vi "Version.vi"(0 "VISA Resource Name":refnum<visa-resource-name>, 11 "error in (no error)":errorcluster) -> (2 "Module 3":string, 3 "Measurement Processor":string, 4 "VISA Resource Name Out":refnum<visa-resource-name>, 6 "I/O Processor":string, 8 "Front Panel Processor":string, 10 "Module 2":string, 13 "Module 1":string, 14 "SCPI Version":string, 15 "error out":errorcluster)   [LabVIEW 2012, in "Agilent 34970.lvlib"]
doc: "This VI queries the HP34970A as well as all its modules for version information."
uses:
  <instrlib>/Agilent 34970/Agilent 34970.lvlib
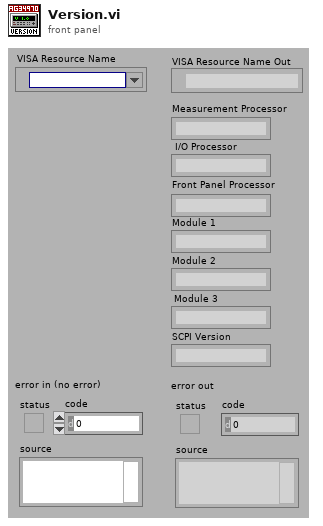
[diagram p1: front panel]
types:
  T1 = cluster{"[0]":string, "[1]":string, "[2]":string, "[3]":string, "[4]":string}
  T2 = cluster{"Output String Array[0]":string, "Output String Array[1]":string, "Output String Array[2]":string}
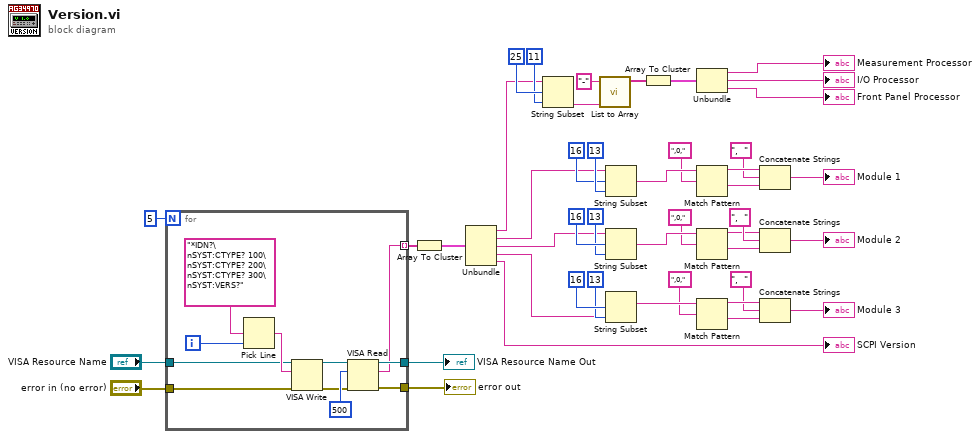
[diagram p0: block diagram]
diagram:
  n1 = for {
    N: 5 -> [_]
    tunnel: [w52] -> w43
    tunnel: [w51] -> w42
    tunnel: "VISA Resource Name" -> [w49]
    tunnel: "error in (no error)" -> [w48]
    tunnel: [w46] -> w7 mode=indexing
    i -> [w55]
    n2 = Pick Line(multi-line string="*IDN?\nSYST:CTYPE? 100\nSYST:CTYPE? 200\nSYST:CTYPE? 300\nSYST:VERS?", line index=w55) -> (output string=w50:string)  [unwired: 1 in]
    n3 = VISA Write(VISA resource name=w49, write buffer=w50, error in (no error)=w48) -> (VISA resource name out=w53:refnum<visa-resource-name>, error out=w47:errorcluster)  [unwired: 1 out]
    n4 = VISA Read(VISA resource name=w53, byte count=u32 500 ("byte count (0)"), error in (no error)=w47) -> (VISA resource name out=w51:refnum<visa-resource-name>, read buffer=w46:string, error out=w52:errorcluster)  [unwired: 1 out]
  }
  "VISA Resource Name Out" <- w42
  "error out" <- w43
  n5 = Array To Cluster(array=w7) -> (cluster=w6:T1)
  n6 = Unbundle(w6) -> ("[0]"=w2:string, "[1]"=w5:string, "[2]"=w4:string, "[3]"=w1:string, "[4]"=→"SCPI Version":string)
  n7 = String Subset(string=w2, offset (0)=25, length (rest)=11 ("length")) -> (substring=w23:string)
  n8 = call <instrlib>:"List to Array.vi"("List (empty)"=w23, "Separator (,)"="-" ("Separator")) -> ("Output String Array"=w41:string[])  [unwired: 8 in, 1 out]
  n9 = String Subset(string=w5, offset (0)=16, length (rest)=13 ("length")) -> (substring=w30:string)
  n10 = String Subset(string=w4, offset (0)=16, length (rest)=13 ("length")) -> (substring=w34:string)
  n11 = String Subset(string=w1, offset (0)=16, length (rest)=13 ("length")) -> (substring=w39:string)
  n12 = Array To Cluster(array=w41) -> (cluster=w22:T2)
  n13 = Unbundle(w22) -> ("Output String Array[0]"=→"Measurement Processor":string, "Output String Array[1]"=→"I/O Processor":string, "Output String Array[2]"=→"Front Panel Processor":string)
  n14 = Match Pattern(string=w30, regular expression=",0," ("string")) -> (before substring=w27:string, after substring=w28:string)  [unwired: 1 in, 2 out]
  n15 = Match Pattern(string=w34, regular expression=",0," ("string")) -> (before substring=w32:string, after substring=w35:string)  [unwired: 1 in, 2 out]
  n16 = Match Pattern(string=w39, regular expression=",0," ("string")) -> (before substring=w37:string, after substring=w40:string)  [unwired: 1 in, 2 out]
  n17 = Concatenate Strings(w27, ",  ", w28) -> (→"Module 1":string)
  n18 = Concatenate Strings(w32, ",  ", w35) -> (→"Module 2":string)
  n19 = Concatenate Strings(w37, ",  ", w40) -> (→"Module 3":string)
